vi "init.vi"(8 "error in (no error)":errorcluster, 11 "ILCTC in":refnum<class "ILCTC.lvclass">) -> (0 "error out":errorcluster, 3 "ILCTC out":refnum<class "ILCTC.lvclass">)   [LabVIEW 2015, in "ILCTC.lvclass"]
uses:
  ILCTC.lvclass
  <userlib>/Common/ILC/Configuration/ILCSerial.ctl
  <userlib>/Common/SerialProtocols/Configuration/SerialConfig.ctl
  <userlib>/Common/SerialProtocols/Configuration/SerialProtocol.ctl
  <userlib>/Common/SerialProtocols/Configuration/ProtocolParameters.ctl
  <userlib>/Common/SerialProtocols/Configuration/SerialMessageParameters.ctl
  <userlib>/Common/ILC/Configuration/ILCADC.ctl
  <userlib>/Common/ILC/Typedefs/ADCSettings.ctl
  <userlib>/Common/ILC/Configuration/InputChannels.ctl
  <userlib>/Common/ILC/Configuration/ScanRate_Hz_MultichannelOptions.ctl
  <userlib>/Common/ILC/ILC/ILC.lvclass/ILC.ctl
  <userlib>/Common/ILC/ILC/ILC.lvclass
  <userlib>/Common/SerialProtocols/SerialProtocols.lvlib
  <userlib>/Common/ILC/Configuration/ILCConfiguration.lvlib
  ConfigurationThisComponent/ConfigurationThisComponent.lvclass
  <userlib>/Common/ILC/Typedefs/ILCTypedefs.lvlib
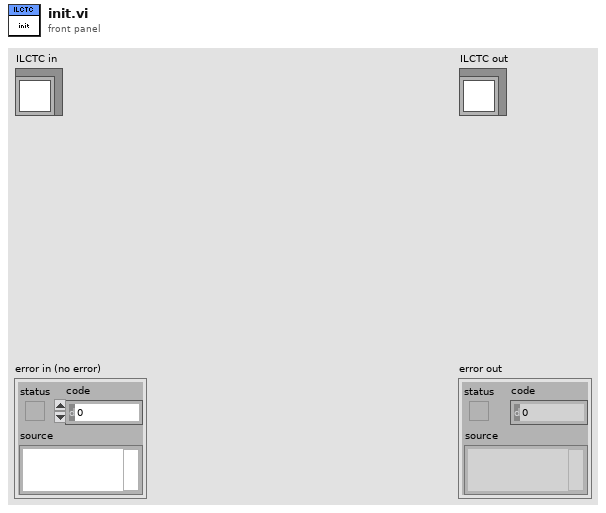
[diagram p1: front panel]
types:
  T1 = typedef "ILCCommon.lvlib/ILCTypedefs.lvlib/ADCSettings.ctl" = cluster{"Input Channels":T2, "Scan Rate (Hz) ":T3, "PGA Gain Coefficient":u8}
  T2 = typedef "ILCCommon.lvlib/ILCConfiguration.lvlib/InputChannels.ctl" = enum16{"Channel 0", "3 Channels", "5 Channels"}
  T3 = typedef "ILCCommon.lvlib/ILCConfiguration.lvlib/ScanRate_Hz_MultichannelOptions.ctl" = enum16{"50", "60", "100", "120", "200", "240", "300", "400", "480", "600", "1200", "2400", "4800"}
  T4 = typedef "ILCCommon.lvlib/ILCConfiguration.lvlib/ILCADC.ctl" = cluster{"Reference Voltage Vref":dbl[unit], "Nominal Input Range in Counts":u32, "Preamplifier Gain":u8, "Conversion Settling Cycles":u16}
  T5 = typedef "ILCCommon.lvlib/ILCConfiguration.lvlib/ILCSerial.ctl" = cluster{"Serial":T6}
  T6 = typedef "SerialProtocols.lvlib/SerialConfig.ctl" = cluster{"Serial Protocol":T7, "Protocol Parameters":T8, "Serial Message Parameters":T9}
  T7 = typedef "SerialProtocols.lvlib/SerialProtocol.ctl" = enum16{"RS232", "RS485", "SerialSimulator"}
  T8 = typedef "SerialProtocols.lvlib/ProtocolParameters.ctl" = cluster{"VISA resource name":refnum<visa-resource-name>, "Baud Rate":u32, "Data Bits":u16, "Parity":enum16{"None", "Odd", "Even", "Mark", "Space"}, "Flow Control":u16, "Stop Bits":u16, "Timeout (ms)":u32}
  T9 = typedef "SerialProtocols.lvlib/SerialMessageParameters.ctl" = cluster{"Byte Count":u32, "Enable Termination Character":bool, "Termination Char":u8}
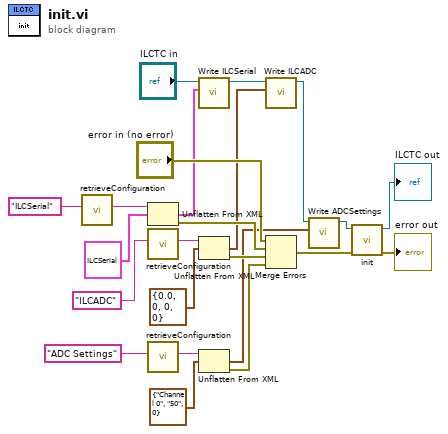
[diagram p0: block diagram]
diagram:
  n1 = call "retrieveConfiguration.vi"("configName"="ILCSerial") -> ("xmlConfig"=w18:string)  [unwired: 8 in, 2 out]
  n2 = Unflatten From XML(xml string=w18, type=T5 {"Serial"={"Serial Protocol"=enum."RS232", "Protocol Parameters"={"VISA resource name"="", "Baud Rate"=0, "Data Bits"=0, "Parity"=enum."None", "Flow Control"=0, "Stop Bits"=0, "Timeout (ms)"=0}, "Serial Message Parameters"={"Byte Count"=0, "Enable Termination Character"=FALSE, "Termination Char"=0}}} ("ILC")) -> (value=w10:T5, error out=w21:errorcluster)  [unwired: 1 in]
  n3 = call "retrieveConfiguration.vi"("configName"="ILCADC") -> ("xmlConfig"=w16:string)  [unwired: 8 in, 2 out]
  n4 = call "retrieveConfiguration.vi"("configName"="ADC Settings") -> ("xmlConfig"=w7:string)  [unwired: 8 in, 2 out]
  n5 = call <userlib>:"Write ILCSerial.vi"("ILC Serial"=w10, "ILC in"="ILCTC in") -> ("ILC out"=w11:refnum<class "ILCTC.lvclass">)  [unwired: 9 in]
  n6 = Unflatten From XML(xml string=w16, type=T4 {"Reference Voltage Vref"=0.0, "Nominal Input Range in Counts"=0, "Preamplifier Gain"=0, "Conversion Settling Cycles"=0} ("ILC ADC")) -> (value=w9:T4, error out=w14:errorcluster)  [unwired: 1 in]
  n7 = Unflatten From XML(xml string=w7, type=T1 {"Input Channels"=enum."Channel 0", "Scan Rate (Hz) "=enum."50", "PGA Gain Coefficient"=0} ("ADC Settings")) -> (value=w2:T1, error out=w1:errorcluster)  [unwired: 1 in]
  n8 = call <userlib>:"Write ILCADC.vi"("ILC ADC"=w9, "ILC in"=w11) -> ("ILC out"=w4:refnum<class "ILCTC.lvclass">)  [unwired: 9 in]
  n9 = Merge Errors("error in (no error)", w21, w14, w1) -> (w8:errorcluster)
  n10 = call <userlib>:"Write ADCSettings.vi"("ADC Settings"=w2, "ILC in"=w4) -> ("ILC out"=w3:refnum<class "ILCTC.lvclass">)  [unwired: 9 in]
  n11 = call-parent "init.vi"("error in (no error)"=w8, "ILC in"=w3) -> ("error out"=→"error out":errorcluster, "ILC out"=→"ILCTC out":refnum<class "ILCTC.lvclass">)  [unwired: 8 in]
